vi "test parse tcp replies.vi"() -> ()   [LabVIEW 2020]
panel:
  out "variable names":string[][](array[string])
  in  "tcp wait all replies":string[](array[string])=["HEX-PL1-1>>50>>xpos nval,-12.000000 nvar,\r\nypos nval,0.000000 nvar,\r\nzpos nval,0.000000 nvar,\r\nuangle nval,0.000000 nvar,\r\nvangle nval,0.300000 nvar,\r\nwangle nval,0.000000 nvar,\r\n", "DDG-AA-ShotCntrl>>50>>Delay.Ch H nval,0.001000000000000 nvar,\r\nDelay.Ch A nval,1.020000000000000 nvar,\r\nDelay.Ch B nval,0.070000000000000 nvar,\r\nDelay.Ch C nval,1.000000000000000 nvar,\r\nDelay.Ch D nval,0.005000000000000 nvar,\r\nDelay.Ch E nval,0.100000000000000 nvar,\r\nDelay.Ch F nval,1.000000000000000 nvar,\r\nDelay.Ch G nval,0.100000000000000 nvar,\r\n", "SVE-LT-Thales>>50>>Thales.DIAG_CU_Power_Amp3_1 nval,327.679000 nvar,\r\nThales.DIAG_CU_Power_Amp2_1 nval,0.500000 nvar,\r\nThales.DIAG_CU_Power_Amp1_1 nval,0.200000 nvar,\r\nThales.DIAG_CU_Power_Preamp_1 nval,-0.500000 nvar,\r\nThales.Spectrum_Amp3_FWHM nval,1.828857 nvar,\r\n", "FW-BELLA-General>>50>>pos.Channel0 nval,2 nvar,\r\npos.Channel1 nval,2 nvar,\r\npos.Channel2 nval,5 nvar,\r\npos.Channel3 nval,5 nvar,\r\npos.Channel4 nval,5 nvar,\r\npos.Channel5 nval,5 nvar,\r\npos.Channel6 nval,6 nvar,\r\npos.Channel7 nval,2 nvar,\r\npos.Channel8 nval,5 nvar,\r\npos.Channel9 nval,6 nvar,\r\npos.Channel10 nval,5 nvar,\r\npos.Channel11 nval,4 nvar,\r\npos.Channel12 nval,2 nvar,\r\n", "STAGE-1BL-Compression>>50>>position nval, nvar,\r\nPosition.Axis 1 nval,9.100000 nvar,\r\nPosition.Axis 2 nval,-14.939500 nvar,\r\nPosition.Axis 3 nval,4.221500 nvar,\r\nPosition.Axis 4 nval,2.090000 nvar,\r\n", "STAGE-HPD-Tel>>50>>position nval,289.000048 nvar,\r\n", "DAQ-AA-1>>50>>Measurements.Analysis1 nval, nvar,\r\nMeasurements.Analysis2 nval,0.002263936542 nvar,\r\n", "DDG-AA-SRS2>>50>>Delay.Ch E nval,0.000262537000000 nvar,\r\nDelay.Ch C nval,0.000262657000000 nvar,\r\nAmplitude.Ch CD nval,4.000000000000000 nvar,\r\nDelay.Ch G nval,0.000261140000000 nvar,\r\n", "DAQ-AA-2>>50>>Measurements.Analysis1 nval,-0.726869377051 nvar,\r\nMeasurements.Analysis2 nval,-0.768258934174 nvar,\r\n", "DAQ-AA-3>>50>>Measurements.Analysis1 nval,0.316289336210 nvar,\r\n", "CAM-HPD-CCD>>50>>centroidx nval,861.778870 nvar,\r\ncentroidy nval,613.786682 nvar,\r\nMaxCounts nval,23.000000 nvar,\r\n2ndmomW0x nval,195.701538 nvar,\r\n2ndmomW0y nval,668.626831 nvar,\r\n2ndmomW0x45 nval,121.923683 nvar,\r\n2ndmomW0y45 nval,119.008621 nvar,\r\nFWHMx nval,1625.000000 nvar,\r\nFWHMy nval,1235.000000 nvar,\r\nMeanCounts nval,1.593041 nvar,\r\nAnalysis nval,on nvar,\r\n", "STAGE-PL1-Smaract>>50>>Position.Channel 3 nval,0.000129 nvar,\r\nPosition.Channel 4 nval,9.000000 nvar,\r\nPosition.Channel 1 nval,0.000129 nvar,\r\nPosition.Channel 5 nval,0.000129 nvar,\r\n", "SPEC-AA-Hamamastsu>>50>>save nval,on nvar,\r\nexposure nval,3.000000 nvar,\r\nMeanWavelength nval,0.000000 nvar,\r\nlambda_r nval,0.000000 nvar,\r\nlambda_b nval,0.000000 nvar,\r\nFWHM nval,0.000000 nvar,\r\nlambda_width (SD) nval,0.000000 nvar,\r\nAverageCountLevel nval,0.000000 nvar,\r\ntrigger nval,off nvar,\r\n", "IP2-targetobs>>50>>exposure nval,0.200000 nvar,\r\nMeanCounts nval, nvar,\r\n", "DDG-AA-SRS0>>50>>delay.Channel_C nval, nvar,\r\nDelay.Ch C nval,0.000000400000000 nvar,\r\nDelay.Ch E nval,0.000261240000000 nvar,\r\n", "MANPAR-BELLA-General>>50>>value1 nval,0.000000000000 nvar,\r\nvalue2 nval,0.000000000000 nvar,\r\nvalue3 nval,3.450000000000 nvar,\r\nvalue4 nval,0.000000000000 nvar,\r\nvalue5 nval,1.000000000000 nvar,\r\nvalue6 nval,0.000000000000 nvar,\r\nvalue7 nval,0.000000000000 nvar,\r\nvalue8 nval,0.000000000000 nvar,\r\n", "IP2-TargetXYZ>>50>>Position.Axis 1 nval,45.000000 nvar,\r\nPosition.Axis 2 nval,-10.829360 nvar,\r\nPosition.Axis 3 nval,190.000000 nvar,\r\n", "CAM-HPD-HolyWedge>>50>>MeanCounts nval, nvar,\r\nMaxCounts nval, nvar,\r\n", "IP2-MCPcam>>50>>centroidx nval,1509.566406 nvar,\r\ncentroidy nval,944.849182 nvar,\r\nMaxCounts nval,3997.000000 nvar,\r\nMeanCounts nval,2169.245605 nvar,\r\n2ndmomW0x45 nval,895.576111 nvar,\r\n2ndmomW0x nval,116.561882 nvar,\r\n2ndmomW0y45 nval,216.802872 nvar,\r\n2ndmomW0y nval,113.743660 nvar,\r\ntrigger nval,on nvar,\r\n", "IP2-modeim>>50>>2ndmomW0x45 nval, nvar,\r\n2ndmomW0x nval, nvar,\r\n2ndmomW0y45 nval, nvar,\r\n2ndmomW0y nval, nvar,\r\ncentroidx nval, nvar,\r\ncentroidy nval, nvar,\r\nexposure nval,0.002000 nvar,\r\nFWHMx nval, nvar,\r\nFWHMy nval, nvar,\r\nMaxCounts nval, nvar,\r\nMaxGUIPixel nval,2000.000000 nvar,\r\n", "IP2-targetscatt>>50>>exposure nval,0.002000 nvar,\r\ncentroidy nval, nvar,\r\ncentroidx nval, nvar,\r\nAnalysis nval,off nvar,\r\n2ndmomW0y nval, nvar,\r\n2ndmomW0y45 nval, nvar,\r\nMaxCounts nval, nvar,\r\n2ndmomW0x nval, nvar,\r\n2ndmomW0x45 nval, nvar,\r\n", "CAM-1BL-M1>>50>>MeanCounts nval, nvar,\r\nexposure nval,0.001000 nvar,\r\n", "SCOPE-AA-LeCroy8254M>>50>>TimeAxis.Time base nval,0.000000500000000 nvar,\r\n", "DateTime>>50>>Timestamp nval,3756531394.448141570 nvar,\r\n", "Rep Rate>>50>>Hz nval,0.493340 nvar,\r\n"]
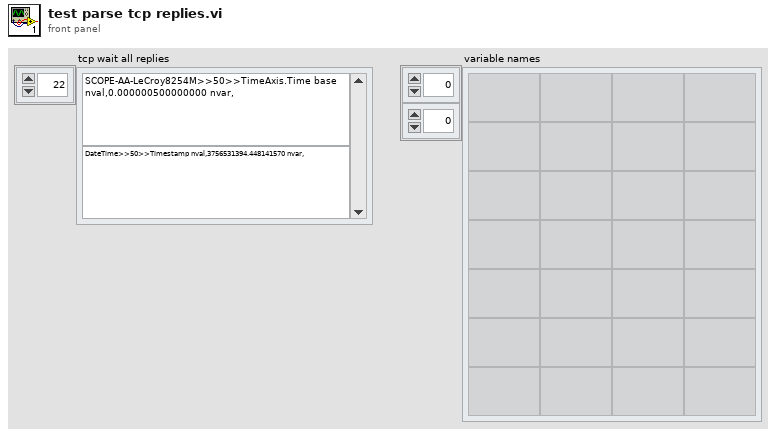
[diagram p1: front panel]
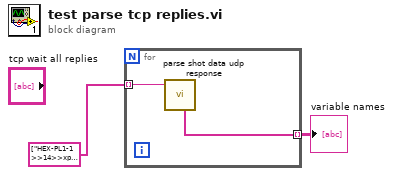
[diagram p0: block diagram]
diagram:
  n1 = for {
    tunnel: string[] ["HEX-PL1-1>>14>>xpos nval,-12.000000 nvar,\r\nypos nval,0.000000 nvar,\r\nzpos nval,0.000000 nvar,\r\nuangle nval,0.000000 nvar,\r\nvangle nval,0.300000 nvar,\r\nwangle nval,0.000000 nvar,\r\n", "DDG-AA-ShotCntrl>>14>>Delay.Ch H nval,0.001000000000000 nvar,\r\nDelay.Ch A nval,1.020000000000000 nvar,\r\nDelay.Ch B nval,0.070000000000000 nvar,\r\nDelay.Ch C nval,1.000000000000000 nvar,\r\nDelay.Ch D nval,0.005000000000000 nvar,\r\nDelay.Ch E nval,0.100000000000000 nvar,\r\nDelay.Ch F nval,1.000000000000000 nvar,\r\nDelay.Ch G nval,0.100000000000000 nvar,\r\n", "SVE-LT-Thales>>14>>Thales.DIAG_CU_Power_Amp3_1 nval,327.679000 nvar,\r\nThales.DIAG_CU_Power_Amp2_1 nval,0.500000 nvar,\r\nThales.DIAG_CU_Power_Amp1_1 nval,0.200000 nvar,\r\nThales.DIAG_CU_Power_Preamp_1 nval,-0.500000 nvar,\r\nThales.Spectrum_Amp3_FWHM nval,1.828857 nvar,\r\n", "FW-BELLA-General>>14>>pos.Channel0 nval,2 nvar,\r\npos.Channel1 nval,2 nvar,\r\npos.Channel2 nval,5 nvar,\r\npos.Channel3 nval,5 nvar,\r\npos.Channel4 nval,5 nvar,\r\npos.Channel5 nval,5 nvar,\r\npos.Channel6 nval,6 nvar,\r\npos.Channel7 nval,2 nvar,\r\npos.Channel8 nval,5 nvar,\r\npos.Channel9 nval,6 nvar,\r\npos.Channel10 nval,5 nvar,\r\npos.Channel11 nval,4 nvar,\r\npos.Channel12 nval,2 nvar,\r\n", "STAGE-1BL-Compression>>14>>position nval, nvar,\r\nPosition.Axis 1 nval,9.100000 nvar,\r\nPosition.Axis 2 nval,-14.939500 nvar,\r\nPosition.Axis 3 nval,4.221500 nvar,\r\nPosition.Axis 4 nval,2.090000 nvar,\r\n", "STAGE-HPD-Tel>>14>>position nval,289.000048 nvar,\r\n", "DAQ-AA-1>>14>>Measurements.Analysis1 nval, nvar,\r\nMeasurements.Analysis2 nval,0.002263936542 nvar,\r\n", "DDG-AA-SRS2>>14>>Delay.Ch E nval,0.000262537000000 nvar,\r\nDelay.Ch C nval,0.000262657000000 nvar,\r\nAmplitude.Ch CD nval,4.000000000000000 nvar,\r\nDelay.Ch G nval,0.000261140000000 nvar,\r\n", "DAQ-AA-2>>14>>Measurements.Analysis1 nval,-0.727714061890 nvar,\r\nMeasurements.Analysis2 nval,-0.768258934174 nvar,\r\n", "DAQ-AA-3>>14>>Measurements.Analysis1 nval,0.316289336210 nvar,\r\n", "CAM-HPD-CCD>>14>>centroidx nval,864.217834 nvar,\r\ncentroidy nval,626.401855 nvar,\r\nMaxCounts nval,22.000000 nvar,\r\n2ndmomW0x nval,NaN nvar,\r\n2ndmomW0y nval,209.968018 nvar,\r\n2ndmomW0x45 nval,117.417702 nvar,\r\n2ndmomW0y45 nval,115.796593 nvar,\r\nFWHMx nval,1625.000000 nvar,\r\nFWHMy nval,1235.000000 nvar,\r\nMeanCounts nval,1.564855 nvar,\r\nAnalysis nval,on nvar,\r\n", "STAGE-PL1-Smaract>>14>>Position.Channel 3 nval,0.000129 nvar,\r\nPosition.Channel 4 nval,8.999997 nvar,\r\nPosition.Channel 1 nval,0.000129 nvar,\r\nPosition.Channel 5 nval,0.000129 nvar,\r\n", "SPEC-AA-Hamamastsu>>14>>save nval,on nvar,\r\nexposure nval,3.000000 nvar,\r\nMeanWavelength nval,0.000000 nvar,\r\nlambda_r nval,0.000000 nvar,\r\nlambda_b nval,0.000000 nvar,\r\nFWHM nval,0.000000 nvar,\r\nlambda_width (SD) nval,0.000000 nvar,\r\nAverageCountLevel nval,0.000000 nvar,\r\ntrigger nval,off nvar,\r\n", "IP2-targetobs>>0>>exposure nval,0.200000 nvar,\r\nMeanCounts nval, nvar,\r\n", "DDG-AA-SRS0>>14>>delay.Channel_C nval, nvar,\r\nDelay.Ch C nval,0.000000400000000 nvar,\r\nDelay.Ch E nval,0.000261240000000 nvar,\r\n", "MANPAR-BELLA-General>>14>>value1 nval,0.000000000000 nvar,\r\nvalue2 nval,0.000000000000 nvar,\r\nvalue3 nval,3.450000000000 nvar,\r\nvalue4 nval,0.000000000000 nvar,\r\nvalue5 nval,1.000000000000 nvar,\r\nvalue6 nval,0.000000000000 nvar,\r\nvalue7 nval,0.000000000000 nvar,\r\nvalue8 nval,0.000000000000 nvar,\r\n", "IP2-TargetXYZ>>14>>Position.Axis 1 nval,45.000000 nvar,\r\nPosition.Axis 2 nval,-10.829360 nvar,\r\nPosition.Axis 3 nval,190.000000 nvar,\r\n", "CAM-HPD-HolyWedge>>14>>MeanCounts nval, nvar,\r\nMaxCounts nval, nvar,\r\n", "IP2-MCPcam>>0>>centroidx nval,1509.347290 nvar,\r\ncentroidy nval,960.451599 nvar,\r\nMaxCounts nval,3997.000000 nvar,\r\nMeanCounts nval,2195.957031 nvar,\r\n2ndmomW0x45 nval,918.957947 nvar,\r\n2ndmomW0x nval,116.394447 nvar,\r\n2ndmomW0y45 nval,203.277267 nvar,\r\n2ndmomW0y nval,124.251183 nvar,\r\ntrigger nval,on nvar,\r\n", "IP2-modeim>>0>>2ndmomW0x45 nval, nvar,\r\n2ndmomW0x nval, nvar,\r\n2ndmomW0y45 nval, nvar,\r\n2ndmomW0y nval, nvar,\r\ncentroidx nval, nvar,\r\ncentroidy nval, nvar,\r\nexposure nval,0.002000 nvar,\r\nFWHMx nval, nvar,\r\nFWHMy nval, nvar,\r\nMaxCounts nval, nvar,\r\nMaxGUIPixel nval,2000.000000 nvar,\r\n", "IP2-targetscatt>>0>>exposure nval,0.002000 nvar,\r\ncentroidy nval, nvar,\r\ncentroidx nval, nvar,\r\nAnalysis nval,off nvar,\r\n2ndmomW0y nval, nvar,\r\n2ndmomW0y45 nval, nvar,\r\nMaxCounts nval, nvar,\r\n2ndmomW0x nval, nvar,\r\n2ndmomW0x45 nval, nvar,\r\n", "CAM-1BL-M1>>14>>MeanCounts nval, nvar,\r\nexposure nval,0.001000 nvar,\r\n", "SCOPE-AA-LeCroy8254M>>14>>TimeAxis.Time base nval,0.000000500000000 nvar,\r\n", "DateTime>>14>>Timestamp nval,3756562452.167526240 nvar,\r\n", "Rep Rate>>14>>Hz nval,0.477555 nvar,\r\n"] ("tcp wait all replies") -> [w4] mode=indexing
    tunnel: [w3] -> w2 mode=indexing
    n2 = call "parse shot data udp response.vi"("ShotData UDP response"=w4) -> ("variable names"=w3:string[])  [unwired: 2 in, 5 out]
  }
  "variable names" <- w2
